vi "SaveProgramData.vi"(8 "Error In":errorcluster, 11 "Prog Data In":T1={"Station"=[], "Sensor List"=[], "Sensor Id"=[], "Parameters"=["PM10", "PM2.5", "ozon", "dwutlenek azotu", "dwutlenek siarki", "benzen", "tlenek węgla"], "Values"=[110, 75, 180, 200, 350, 21, 15]}) -> (0 "Error Out":errorcluster, 3 "Prog Data Out":T1={"Station"=[], "Sensor List"=[], "Sensor Id"=[], "Parameters"=["PM10", "PM2.5", "ozon", "dwutlenek azotu", "dwutlenek siarki", "benzen", "tlenek węgla"], "Values"=[110, 75, 180, 200, 350, 21, 15]})   [LabVIEW 2020]
doc: "This VI save program data in Prog Data cluster format."
uses:
  Ctrls/ProgData.ctl
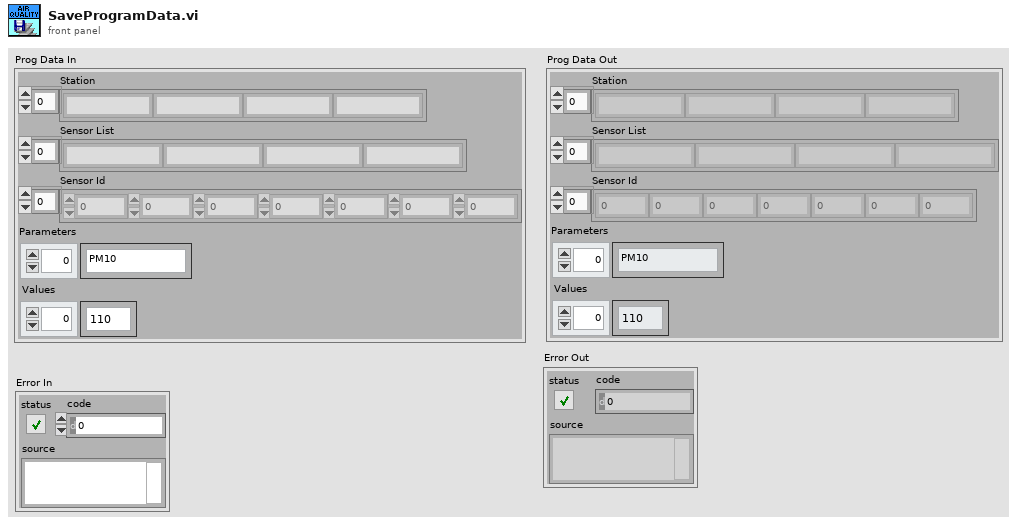
[diagram p1: front panel]
types:
  T1 = typedef "ProgData.ctl" = cluster{"Station":string[], "Sensor List":string[], "Sensor Id":dbl[], "Parameters":string[], "Values":i32[]}
  T2 = enum16{"open", "replace", "create", "open or create", "replace or create", "replace or create with confirmation"}
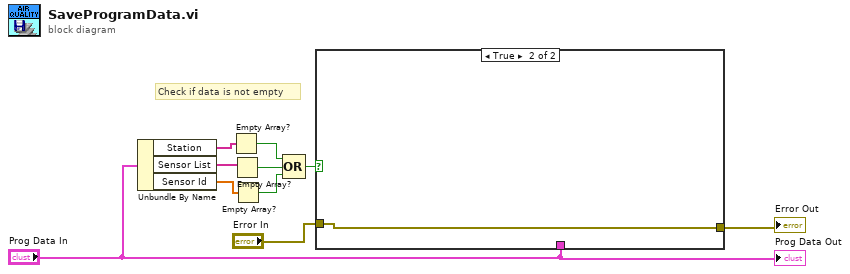
[diagram p0: block diagram]
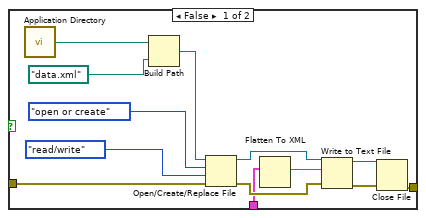
[diagram p2: hidden frame]
diagram:
  # "Check if data is not empty"
  n1 = Unbundle By Name("Prog Data In") -> ("Station"=w6:string[], "Sensor List"=w4:string[], "Sensor Id"=w3:dbl[])
  n2 = Empty Array?(array=w6) -> (empty?=w5:bool)
  n3 = Empty Array?(array=w4) -> (empty?=w2:bool)
  n4 = Empty Array?(array=w3) -> (empty?=w1:bool)
  n5 = Compound Arithmetic op=OR(w5, w2, w1) -> (w8:bool)
  n6 = case shown="True" w8 {
    tunnel: [w13 w24] -> w10
    tunnel: "Prog Data In" -> [w12 _]
    tunnel: "Error In" -> [w11 w24]
    frame False {
      n7 = call <vilib>:"Application Directory.vi"() -> ("Application Directory"=w20:path)
      n8 = Build Path(base path=w20, name or relative path=path "data.xml") -> (appended path=w19:path)
      n9 = Open/Create/Replace File(file path (use dialog)=w19, error in=w11, operation (0:open)=T2."open or create", access (0:read/write)=enum16{"read/write", "read-only", "write-only"}."read/write") -> (refnum out=w18:refnum<file>, error out=w17:errorcluster)  [unwired: 2 in, 1 out]
      n10 = Flatten To XML(6:w12) -> (2:w16:string)
      n11 = Write to Text File(file (use dialog)=w18, text=w16, error in=w17) -> (refnum out=w14:refnum<file>, error out=w15:errorcluster)  [unwired: 1 in, 1 out]
      n12 = Close File(refnum=w14, error in=w15) -> (error out=w13:errorcluster)  [unwired: 1 out]
    }
    frame True {
    }
  }
  "Error Out" <- w10
  "Prog Data Out" <- "Prog Data In"
